vi "Test - 2.vi"() -> ()   [LabVIEW 2013]
uses:
  Channel/Ctls/Dimensions.ctl
  Item/Item.lvclass
  Section/Section.lvclass
  Channel/Channel.lvclass
  Generic/Generic.lvclass
panel:
  out "Values":variant[](array[variant])
  out "Property Names":string[](array[string])
  out "Faultable":bool
  out "Dimensions":T1={"Row"=1, "Column"=1}
  out "replaced":bool
  out "found":bool
  out "Value":variant
  out "PathName 4":string
  out "PathName 3":string
  out "PathName 2":string
  out "Name":string
  out "错误输出":errorcluster
  out "PathName":string
  out "Modified":bool
  out "ClassName":string
  out "ClassID":u32
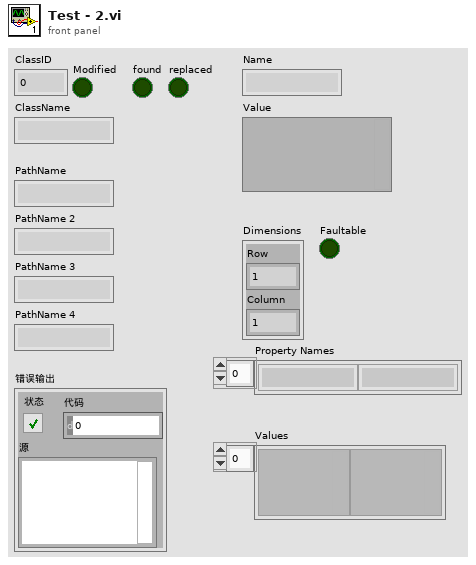
[diagram p1: front panel]
types:
  T1 = typedef "Hierarchy Framework.lvlib/Channel.lvclass/Dimensions.ctl" = cluster{"Row":i32, "Column":i32}
  T2 = typedef "Framework.lvlib/Channel.lvclass/Dimensions.ctl" = cluster{"Row":i32, "Column":i32}
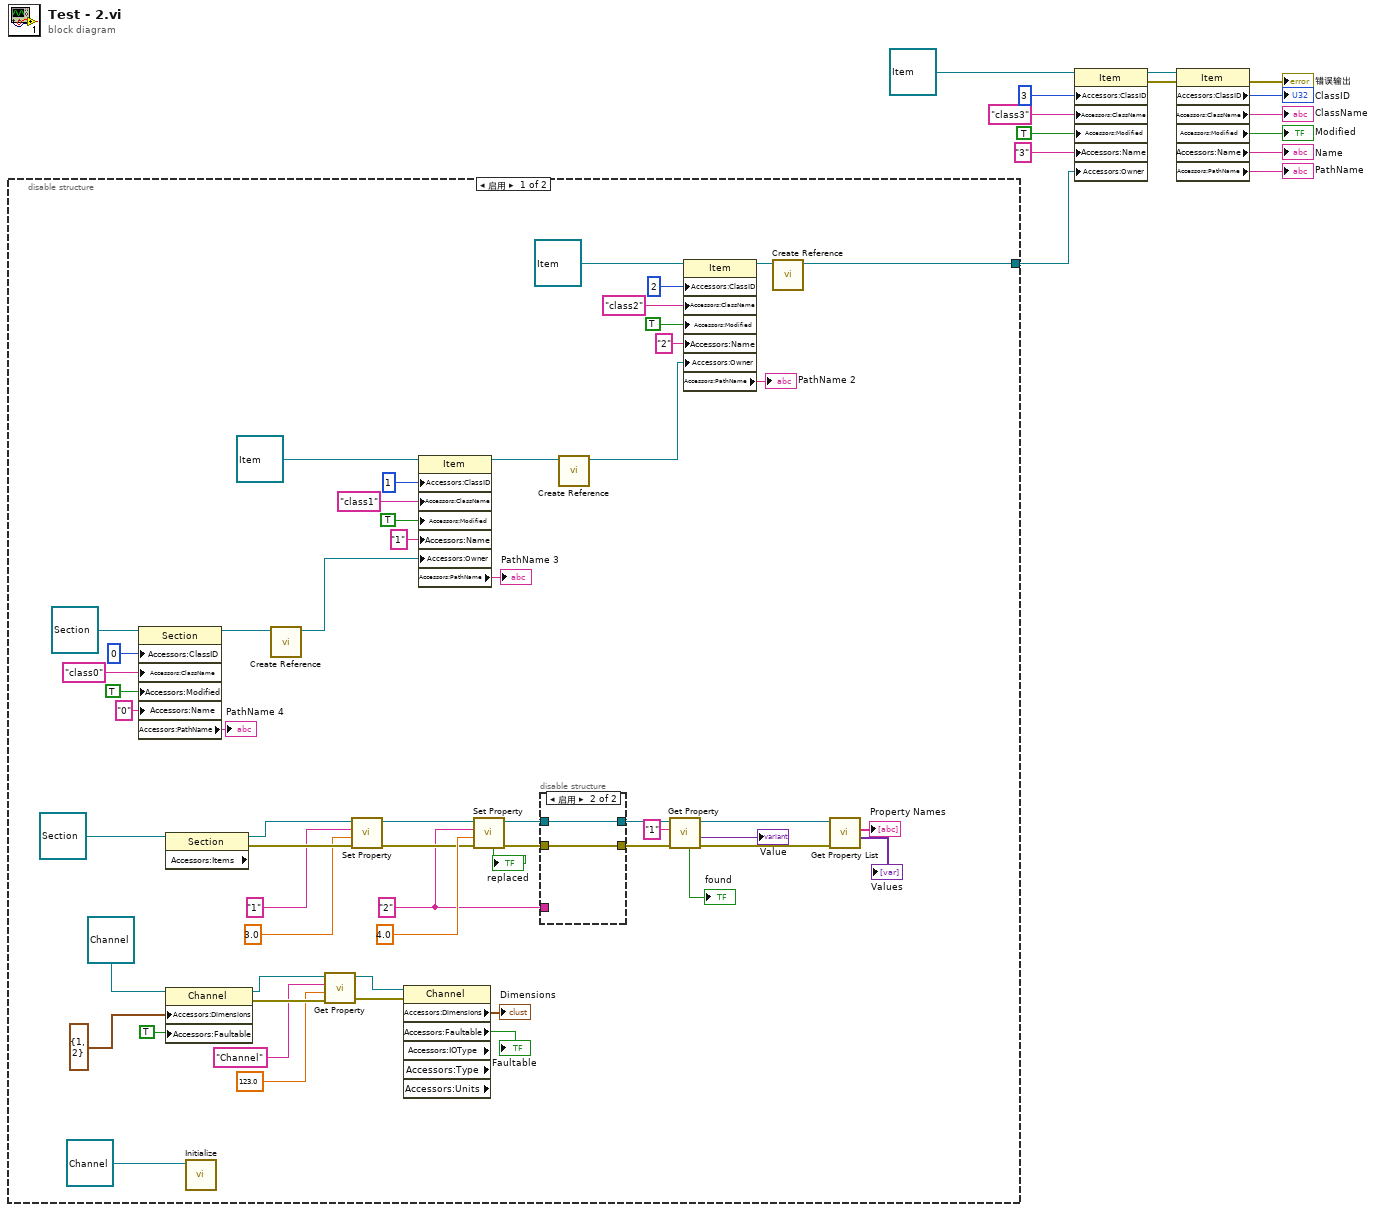
[diagram p0: block diagram]
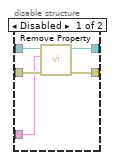
[diagram p2: hidden frame]
diagram:
  n1 = disable-structure shown="启用" {
    disable-tunnel: [w31 _] -> w4
    frame Enabled {
      w44 = "2" ("Tag")
      n2 = property class="Section"(reference=refnum<class "Section.lvclass"> refnum ("Framework.lvlib:Section"), "Accessors:ClassID"=u32 0 ("ClassID"), "Accessors:ClassName"="class0" ("ClassName"), "Accessors:Modified"=TRUE ("Modified"), "Accessors:Name"="0" ("Name")) -> (reference out=w35:refnum<class "Section.lvclass">, "Accessors:PathName"=→"PathName 4":string)  [unwired: 1 in, 1 out]
      n3 = property class="Section" props=["Accessors:Items"](reference=refnum<class "Section.lvclass"> refnum ("Framework.lvlib:Section")) -> (reference out=w56:refnum<class "Section.lvclass">, error out=w55:errorcluster)  [unwired: 1 in, 1 out]
      n4 = property class="Channel"(reference=refnum<class "Channel.lvclass"> refnum ("Framework.lvlib:Channel"), "Accessors:Dimensions"=T1 {"Row"=1, "Column"=2} ("Dimensions"), "Accessors:Faultable"=TRUE ("Faultable")) -> (reference out=w43:refnum<class "Channel.lvclass">, error out=w42:errorcluster)  [unwired: 1 in]
      n5 = call-dynamic "Initialize.vi"("Channel输入"=refnum<class "Channel.lvclass"> refnum ("Framework.lvlib:Channel")) -> ()  [unwired: 9 in, 2 out]
      n6 = call "Create Reference.vi"("Generic"=w35) -> ("Generic Reference"=w30:refnum<data-value>)  [unwired: 9 in, 1 out]
      n7 = call-dynamic "Get Property.vi"("error in (no error)"=w42, "Default Value"=123.0, "Property Name"="Channel" ("Tag"), "Item输入"=w43) -> ("error out"=w40:errorcluster, "Item输出"=w41:refnum<class "Channel.lvclass">)  [unwired: 4 in, 2 out]
      n8 = call-dynamic "Set Property.vi"("error in (no error)"=w55, "Value"=3.0, "Property Name"="1" ("Tag"), "Item输入"=w56) -> ("error out"=w49:errorcluster, "Item输出"=w50:refnum<class "Section.lvclass">)  [unwired: 5 in, 1 out]
      n9 = property class="Channel" props=["Accessors:Dimensions", "Accessors:Faultable", "Accessors:IOType", "Accessors:Type", "Accessors:Units"](reference=w41, error in=w40) -> ("Accessors:Dimensions"=→"Dimensions":T2, "Accessors:Faultable"=→"Faultable":bool)  [unwired: 5 out]
      n10 = property class="Item"(reference=refnum<class "Item.lvclass"> refnum ("Framework.lvlib:Item"), "Accessors:ClassID"=u32 1 ("ClassID"), "Accessors:ClassName"="class1" ("ClassName"), "Accessors:Modified"=TRUE ("Modified"), "Accessors:Name"="1" ("Name"), "Accessors:Owner"=w30) -> (reference out=w33:refnum<class "Item.lvclass">, "Accessors:PathName"=→"PathName 3":string)  [unwired: 1 in, 1 out]
      n11 = call-dynamic "Set Property.vi"("error in (no error)"=w49, "Value"=4.0, "Property Name"=w44, "Item输入"=w50) -> ("error out"=w47:errorcluster, "Item输出"=w48:refnum<class "Section.lvclass">, "replaced"=→"replaced":bool)  [unwired: 5 in]
      n12 = disable-structure shown="启用" {
        disable-tunnel: w48 -> [w76 w78]
        disable-tunnel: w47 -> [w75 w77]
        disable-tunnel: [w74 w78] -> w46
        disable-tunnel: [w73 w77] -> w45
        disable-tunnel: w44 -> [w72 _]
        frame Disabled {
          n13 = call-dynamic "Remove Property.vi"("error in (no error)"=w75, "Property Name"=w72, "Item输入"=w76) -> ("error out"=w73:errorcluster, "Item输出"=w74:refnum<class "Section.lvclass">)  [unwired: 6 in, 1 out]
        }
        frame Enabled {
        }
      }
      n14 = call "Create Reference.vi"("Generic"=w33) -> ("Generic Reference"=w34:refnum<data-value>)  [unwired: 9 in, 1 out]
      n15 = call-dynamic "Get Property.vi"("error in (no error)"=w45, "Property Name"="1" ("Tag"), "Item输入"=w46) -> ("error out"=w19:errorcluster, "Value"=→"Value":variant, "Item输出"=w20:refnum<class "Section.lvclass">, "found"=→"found":bool)  [unwired: 5 in]
      n16 = property class="Item"(reference=refnum<class "Item.lvclass"> refnum ("Framework.lvlib:Item"), "Accessors:ClassID"=u32 2 ("ClassID"), "Accessors:ClassName"="class2" ("ClassName"), "Accessors:Modified"=TRUE ("Modified"), "Accessors:Name"="2" ("Name"), "Accessors:Owner"=w34) -> (reference out=w32:refnum<class "Item.lvclass">, "Accessors:PathName"=→"PathName 2":string)  [unwired: 1 in, 1 out]
      n17 = call "Create Reference.vi"("Generic"=w32) -> ("Generic Reference"=w31:refnum<data-value>)  [unwired: 9 in, 1 out]
      n18 = call-dynamic "Get Property List.vi"("error in (no error)"=w19, "Item输入"=w20) -> ("Values"=→"Values":variant[], "Property Names"=→"Property Names":string[])  [unwired: 6 in, 2 out]
    }
    frame Disabled {
    }
  }
  n19 = property class="Item"(reference=refnum<class "Item.lvclass"> refnum ("Framework.lvlib:Item"), "Accessors:ClassID"=u32 3 ("ClassID"), "Accessors:ClassName"="class3" ("ClassName"), "Accessors:Modified"=TRUE ("Modified"), "Accessors:Name"="3" ("Name"), "Accessors:Owner"=w4) -> (reference out=w8:refnum<class "Item.lvclass">, error out=w6:errorcluster)  [unwired: 1 in]
  n20 = property class="Item"(reference=w8, error in=w6) -> (error out=→"错误输出":errorcluster, "Accessors:ClassID"=→"ClassID":u32, "Accessors:ClassName"=→"ClassName":string, "Accessors:Modified"=→"Modified":bool, "Accessors:Name"=→"Name":string, "Accessors:PathName"=→"PathName":string)  [unwired: 1 out]
